vi "aft_Compute_FWL.vi"(11 "fixed-point configurations":T3) -> (0 "delta":cluster{dbl, dbl, dbl, dbl}, 1 "min":T1, 2 "max":T4, 3 "fwl out":T2)   [LabVIEW 2017, in "NI_AdaptiveFilter.lvlib"]
uses:
  <vilib>/addons/Adaptive Filters/NI_AdaptiveFilter.lvlib
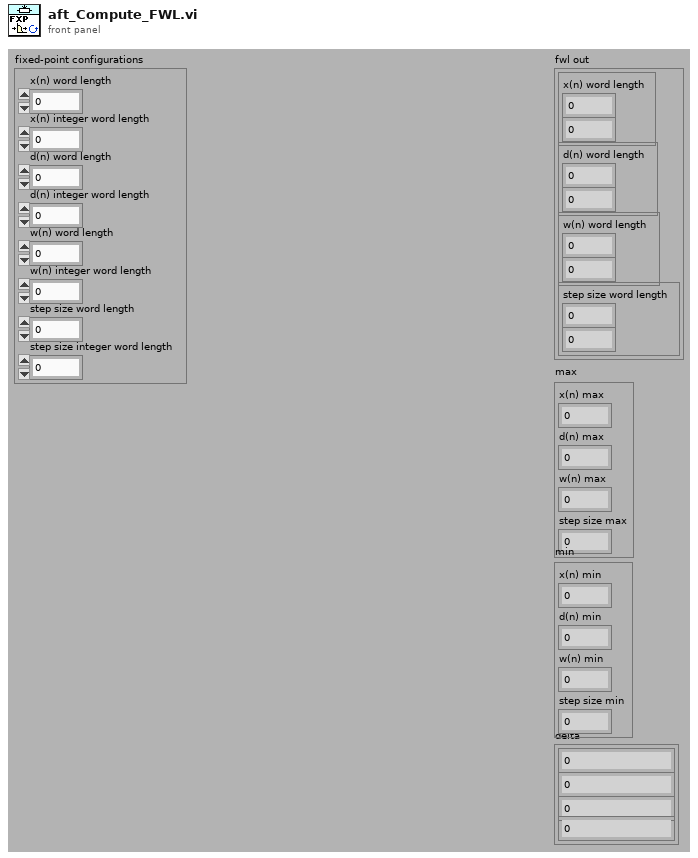
[diagram p1: front panel]
types:
  T1 = cluster{"x(n) min":dbl, "d(n) min":dbl, "w(n) min":dbl, "step size min":dbl}
  T2 = cluster{cluster{"x(n) word length":i32, i32}, cluster{"d(n) word length":i32, i32}, cluster{"w(n) word length":i32, i32}, cluster{"step size word length":i32, i32}}
  T3 = cluster{"x(n) word length":i32, "x(n) integer word length":i32, "d(n) word length":i32, "d(n) integer word length":i32, "w(n) word length":i32, "w(n) integer word length":i32, "step size word length":i32, "step size integer word length":i32}
  T4 = cluster{"x(n) max":dbl, "d(n) max":dbl, "w(n) max":dbl, "step size max":dbl}
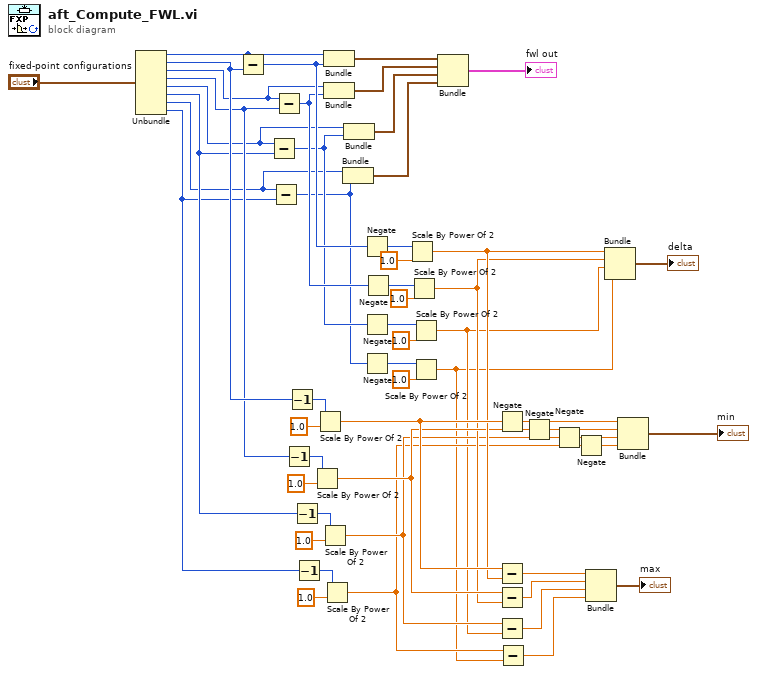
[diagram p0: block diagram]
diagram:
  n1 = Unbundle("fixed-point configurations") -> ("x(n) word length"=w26:i32, "x(n) integer word length"=w25:i32, "d(n) word length"=w24:i32, "d(n) integer word length"=w23:i32, "w(n) word length"=w22:i32, "w(n) integer word length"=w21:i32, "step size word length"=w20:i32, "step size integer word length"=w19:i32)
  n2 = Subtract(x=w26, y=w25) -> (x-y=w43:i32)
  n3 = Subtract(x=w22, y=w21) -> (x-y=w41:i32)
  n4 = Subtract(x=w20, y=w19) -> (x-y=w30:i32)
  n5 = Subtract(x=w24, y=w23) -> (x-y=w42:i32)
  n6 = Decrement(x=w23) -> (x-1=w47:i32)
  n7 = Decrement(x=w25) -> (x-1=w49:i32)
  n8 = Decrement(x=w21) -> (x-1=w45:i32)
  n9 = Decrement(x=w19) -> (x-1=w29:i32)
  n10 = Scale By Power Of 2(n=w47, x=1.0) -> (x*2^n=w10:dbl)
  n11 = Scale By Power Of 2(n=w49, x=1.0) -> (x*2^n=w12:dbl)
  n12 = Scale By Power Of 2(n=w45, x=1.0) -> (x*2^n=w8:dbl)
  n13 = Scale By Power Of 2(n=w29, x=1.0) -> (x*2^n=w7:dbl)
  n14 = Bundle("x(n) word length"=w26, w43) -> (w53:cluster{"x(n) word length":i32, i32})  [unwired: 1 out]
  n15 = Bundle("d(n) word length"=w24, w42) -> (w52:cluster{"d(n) word length":i32, i32})  [unwired: 1 out]
  n16 = Bundle("step size word length"=w20, w30) -> (w34:cluster{"step size word length":i32, i32})  [unwired: 1 out]
  n17 = Bundle("w(n) word length"=w22, w41) -> (w51:cluster{"w(n) word length":i32, i32})  [unwired: 1 out]
  n18 = Negate(x=w43) -> (-x=w40:i32)
  n19 = Negate(x=w41) -> (-x=w31:i32)
  n20 = Negate(x=w30) -> (-x=w33:i32)
  n21 = Negate(x=w42) -> (-x=w37:i32)
  n22 = Scale By Power Of 2(n=w40, x=1.0) -> (x*2^n=w11:dbl)
  n23 = Scale By Power Of 2(n=w37, x=1.0) -> (x*2^n=w9:dbl)
  n24 = Scale By Power Of 2(n=w31, x=1.0) -> (x*2^n=w6:dbl)
  n25 = Scale By Power Of 2(n=w33, x=1.0) -> (x*2^n=w5:dbl)
  n26 = Bundle(w53, w52, w51, w34) -> (→"fwl out":T2)  [unwired: 1 out]
  n27 = Negate(x=w12) -> (-x=w17:dbl)
  n28 = Subtract(x=w12, y=w11) -> (x-y=w4:dbl)
  n29 = Subtract(x=w10, y=w9) -> (x-y=w3:dbl)
  n30 = Subtract(x=w8, y=w6) -> (x-y=w2:dbl)
  n31 = Subtract(x=w7, y=w5) -> (x-y=w1:dbl)
  n32 = Negate(x=w10) -> (-x=w16:dbl)
  n33 = Negate(x=w8) -> (-x=w15:dbl)
  n34 = Negate(x=w7) -> (-x=w14:dbl)
  n35 = Bundle(w4, w3, w2, w1) -> (→"max":cluster{dbl, dbl, dbl, dbl})  [unwired: 1 out]
  n36 = Bundle(w11, w9, w6, w5) -> (→"delta":cluster{dbl, dbl, dbl, dbl})  [unwired: 1 out]
  n37 = Bundle(w17, w16, w15, w14) -> (→"min":cluster{dbl, dbl, dbl, dbl})  [unwired: 1 out]
